vi "KEB Trampa to Accel.vi"(10 "t rampa s":dbl, 11 "rpm max":dbl) -> (3 "upper limit":dbl)   [LabVIEW 2019]
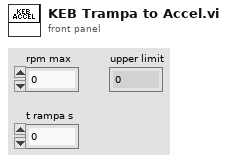
[diagram p1: front panel]
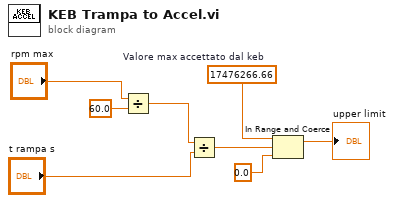
[diagram p0: block diagram]
diagram:
  w7 = 17476266.66  # Valore max accettato dal keb
  n1 = Divide(x="rpm max", y=60.0) -> (x/y=w3:dbl)
  n2 = Divide(x=w3, y="t rampa s") -> (x/y=w5:dbl)
  n3 = In Range and Coerce(upper limit=w7, x=w5, lower limit=0.0) -> (coerced(x)=→"upper limit":dbl)  [unwired: 1 out]
